vi "ISMBUS_DecodeErrorStates.vi"(8 "Fehler (Eingang - kein Fehler)":errorcluster, 10 "Location":string, 11 "ISMBUS_Error State":i32) -> (0 "Fehler (Ausgang)":errorcluster)   [LabVIEW 2016]
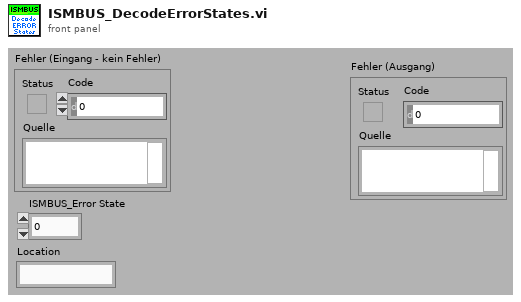
[diagram p1: front panel]
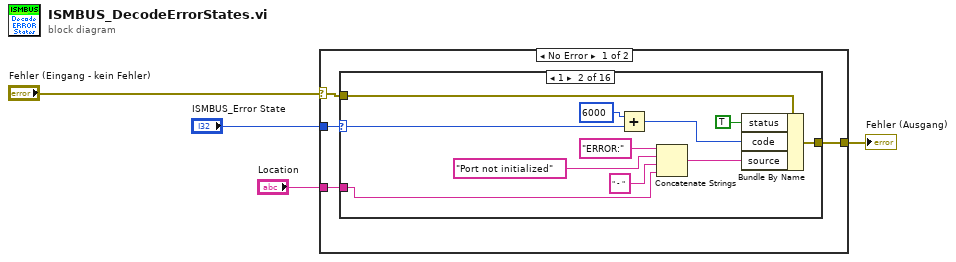
[diagram p0: block diagram]
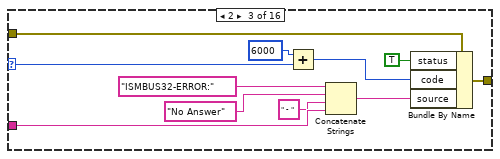
[diagram p3: hidden frame]
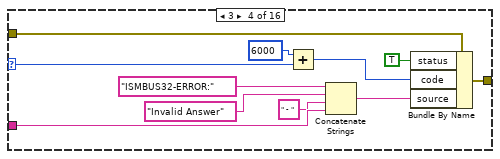
[diagram p4: hidden frame]
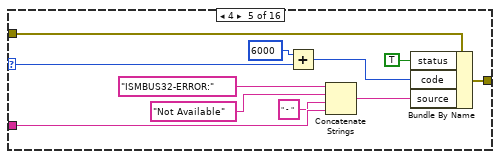
[diagram p5: hidden frame]
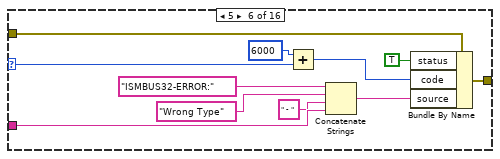
[diagram p6: hidden frame]
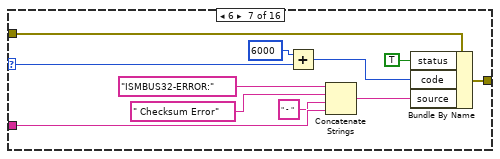
[diagram p7: hidden frame]
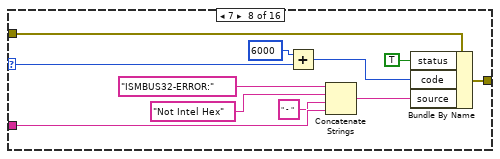
[diagram p8: hidden frame]
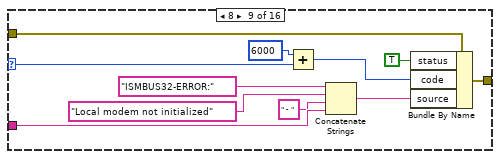
[diagram p9: hidden frame]
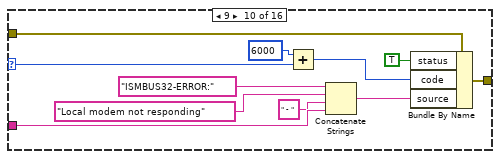
[diagram p10: hidden frame]
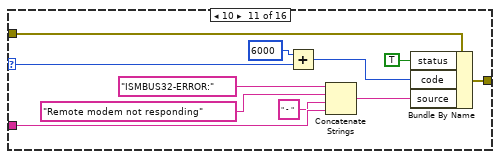
[diagram p11: hidden frame]
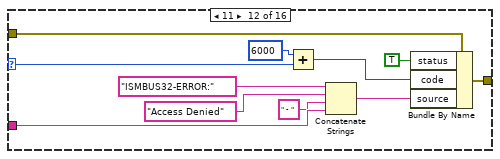
[diagram p12: hidden frame]
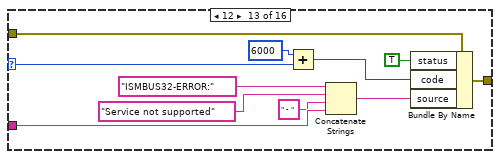
[diagram p13: hidden frame]
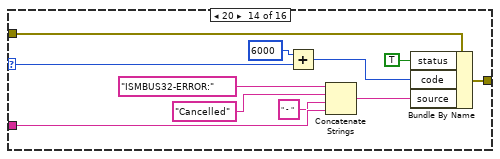
[diagram p14: hidden frame]
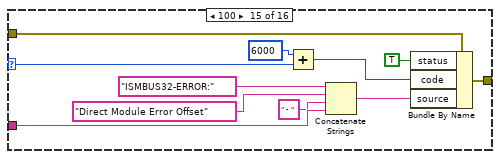
[diagram p15: hidden frame]
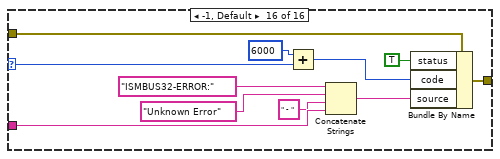
[diagram p16: hidden frame]
diagram:
  n1 = case shown="No Error" "Fehler (Eingang - kein Fehler)" {
    selector: "Fehler (Eingang - kein Fehler)" -> [w7 w175]
    tunnel: [w6 w175] -> w3
    tunnel: "ISMBUS_Error State" -> [w8 _]
    tunnel: "Location" -> [w5 _]
    frame No Error {
      n2 = case shown="1" w8 {
        selector: w8 -> [_ w16 w27 w38 w49 w60 w71 w82 w93 w104 w115 w126 w137 w148 w159 w170]
        tunnel: w7 -> [w9 w19 w30 w41 w52 w63 w74 w85 w96 w107 w118 w129 w140 w151 w162 w173]
        tunnel: [w9 w20 w31 w42 w53 w64 w75 w86 w97 w108 w119 w130 w141 w152 w163 w174] -> w6
        tunnel: w5 -> [_ w13 w24 w35 w46 w57 w68 w79 w90 w101 w112 w123 w134 w145 w156 w167]
        frame 0 {
          # "No ERROR!"
        }
        frame 1 {
          n3 = Add(x=6000, y=w16) -> (x+y=w15:i32)
          n4 = Concatenate Strings("ERROR:" ("String"), "Port not initialized" ("String"), " - " ("String"), w13) -> (w14:string)
          n5 = Bundle By Name(cluster=w19, "status"=TRUE, "code"=w15, "source"=w14) -> (w20:errorcluster)
        }
        frame 2 {
          n6 = Add(x=6000, y=w27) -> (x+y=w26:i32)
          n7 = Concatenate Strings("ISMBUS32-ERROR:" ("String"), "No Answer" ("String"), " - " ("String"), w24) -> (w25:string)
          n8 = Bundle By Name(cluster=w30, "status"=TRUE, "code"=w26, "source"=w25) -> (w31:errorcluster)
        }
        frame 3 {
          n9 = Add(x=6000, y=w38) -> (x+y=w37:i32)
          n10 = Concatenate Strings("ISMBUS32-ERROR:" ("String"), "Invalid Answer" ("String"), " - " ("String"), w35) -> (w36:string)
          n11 = Bundle By Name(cluster=w41, "status"=TRUE, "code"=w37, "source"=w36) -> (w42:errorcluster)
        }
        frame 4 {
          n12 = Add(x=6000, y=w49) -> (x+y=w48:i32)
          n13 = Concatenate Strings("ISMBUS32-ERROR:" ("String"), "Not Available" ("String"), " - " ("String"), w46) -> (w47:string)
          n14 = Bundle By Name(cluster=w52, "status"=TRUE, "code"=w48, "source"=w47) -> (w53:errorcluster)
        }
        frame 5 {
          n15 = Add(x=6000, y=w60) -> (x+y=w59:i32)
          n16 = Concatenate Strings("ISMBUS32-ERROR:" ("String"), "Wrong Type" ("String"), " - " ("String"), w57) -> (w58:string)
          n17 = Bundle By Name(cluster=w63, "status"=TRUE, "code"=w59, "source"=w58) -> (w64:errorcluster)
        }
        frame 6 {
          n18 = Add(x=6000, y=w71) -> (x+y=w70:i32)
          n19 = Concatenate Strings("ISMBUS32-ERROR:" ("String"), " Checksum Error" ("String"), " - " ("String"), w68) -> (w69:string)
          n20 = Bundle By Name(cluster=w74, "status"=TRUE, "code"=w70, "source"=w69) -> (w75:errorcluster)
        }
        frame 7 {
          n21 = Add(x=6000, y=w82) -> (x+y=w81:i32)
          n22 = Concatenate Strings("ISMBUS32-ERROR:" ("String"), "Not Intel Hex" ("String"), " - " ("String"), w79) -> (w80:string)
          n23 = Bundle By Name(cluster=w85, "status"=TRUE, "code"=w81, "source"=w80) -> (w86:errorcluster)
        }
        frame 8 {
          n24 = Add(x=6000, y=w93) -> (x+y=w92:i32)
          n25 = Concatenate Strings("ISMBUS32-ERROR:" ("String"), "Local modem not initialized" ("String"), " - " ("String"), w90) -> (w91:string)
          n26 = Bundle By Name(cluster=w96, "status"=TRUE, "code"=w92, "source"=w91) -> (w97:errorcluster)
        }
        frame 9 {
          n27 = Add(x=6000, y=w104) -> (x+y=w103:i32)
          n28 = Concatenate Strings("ISMBUS32-ERROR:" ("String"), "Local modem not responding" ("String"), " - " ("String"), w101) -> (w102:string)
          n29 = Bundle By Name(cluster=w107, "status"=TRUE, "code"=w103, "source"=w102) -> (w108:errorcluster)
        }
        frame 10 {
          n30 = Add(x=6000, y=w115) -> (x+y=w114:i32)
          n31 = Concatenate Strings("ISMBUS32-ERROR:" ("String"), "Remote modem not responding" ("String"), " - " ("String"), w112) -> (w113:string)
          n32 = Bundle By Name(cluster=w118, "status"=TRUE, "code"=w114, "source"=w113) -> (w119:errorcluster)
        }
        frame 11 {
          n33 = Add(x=6000, y=w126) -> (x+y=w125:i32)
          n34 = Concatenate Strings("ISMBUS32-ERROR:" ("String"), "Access Denied" ("String"), " - " ("String"), w123) -> (w124:string)
          n35 = Bundle By Name(cluster=w129, "status"=TRUE, "code"=w125, "source"=w124) -> (w130:errorcluster)
        }
        frame 12 {
          n36 = Add(x=6000, y=w137) -> (x+y=w136:i32)
          n37 = Concatenate Strings("ISMBUS32-ERROR:" ("String"), "Service not supported" ("String"), " - " ("String"), w134) -> (w135:string)
          n38 = Bundle By Name(cluster=w140, "status"=TRUE, "code"=w136, "source"=w135) -> (w141:errorcluster)
        }
        frame 20 {
          n39 = Add(x=6000, y=w148) -> (x+y=w147:i32)
          n40 = Concatenate Strings("ISMBUS32-ERROR:" ("String"), "Cancelled" ("String"), " - " ("String"), w145) -> (w146:string)
          n41 = Bundle By Name(cluster=w151, "status"=TRUE, "code"=w147, "source"=w146) -> (w152:errorcluster)
        }
        frame 100 {
          n42 = Add(x=6000, y=w159) -> (x+y=w158:i32)
          n43 = Concatenate Strings("ISMBUS32-ERROR:" ("String"), "Direct Module Error Offset" ("String"), " - " ("String"), w156) -> (w157:string)
          n44 = Bundle By Name(cluster=w162, "status"=TRUE, "code"=w158, "source"=w157) -> (w163:errorcluster)
        }
        frame -1, Default {
          n45 = Add(x=6000, y=w170) -> (x+y=w169:i32)
          n46 = Concatenate Strings("ISMBUS32-ERROR:" ("String"), "Unknown Error" ("String"), " - " ("String"), w167) -> (w168:string)
          n47 = Bundle By Name(cluster=w173, "status"=TRUE, "code"=w169, "source"=w168) -> (w174:errorcluster)
        }
      }
    }
    frame Error {
    }
  }
  "Fehler (Ausgang)" <- w3
